vi "Type Info.vi"(11 "Caraya Item in":refnum<class "Caraya Item.lvclass">) -> (1 "Description":string, 2 "Pretty Name":string, 3 "Type":string)   [LabVIEW 2019, in "Caraya Library.lvlib" / "Caraya Item.lvclass"]
doc: "Returns Type information about the solution item.\n----\nCopyright: MGI 2017\nAuthor: Derek Trepanier"
uses:
  Caraya Item.lvclass
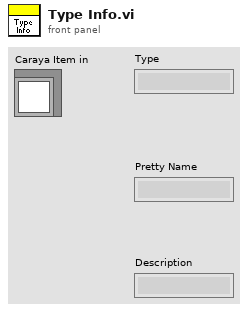
[diagram p1: front panel]
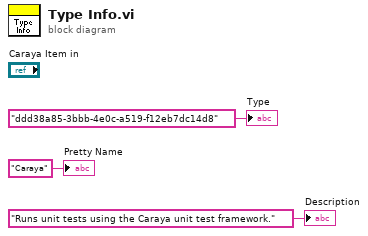
[diagram p0: block diagram]
diagram:
  "Pretty Name" <- "Caraya" ("Pretty Name")
  "Description" <- "Runs unit tests using the Caraya unit test framework." ("Description")
  "Type" <- "ddd38a85-3bbb-4e0c-a519-f12eb7dc14d8" ("Type")
